vi "GetSWRevision.vi"(11 "File Path Control":path caption="File Path Control (leave blank to use Constants_Global value of EnFlo SW Folder)") -> (0 "Brief Output":string, 2 "localStatus":string, 3 "Revision":string)   [LabVIEW 2022 SP3]
doc: "This VI uses the system's installed svn (subversion) software to return the revision number of the selected folder. Leaving the selected folder blank will use the global value of \"EnFlo SW Folder\".\nThe \"Overall Revision\" is the highest revision number in the entire hierarchy, recursing upwards as well as downwards- in other words, the revision which was checked out. The \"This Folder\" data is specific to the last changes to the selected folder."
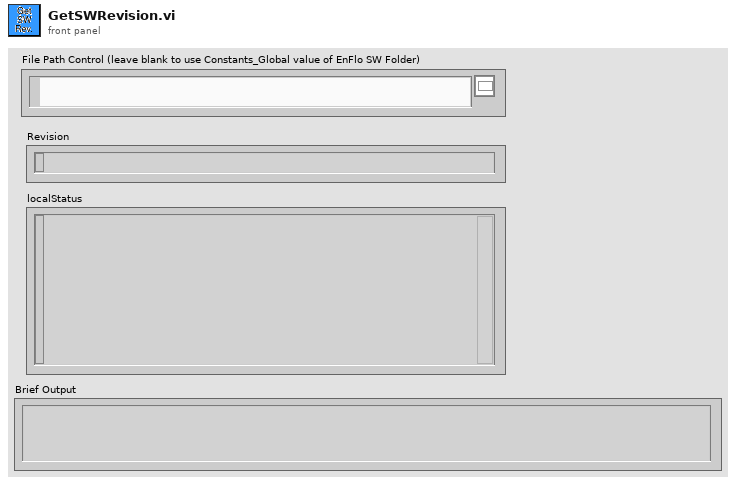
[diagram p1: front panel]
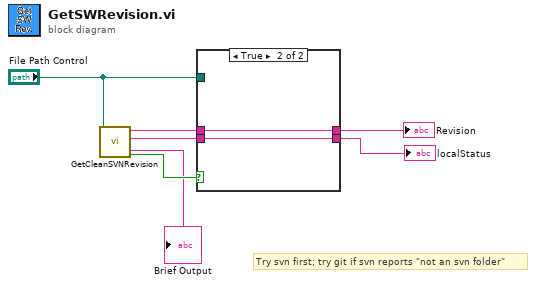
[diagram p0: block diagram]
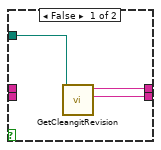
[diagram p2: hidden frame]
diagram:
  # "Try svn first; try git if svn reports \"not an svn folder\""
  n1 = call "GetCleanSVNRevision.vi"("File Path Control"="File Path Control") -> ("isSVN"=w5:bool, "svnDetails"=w7:string, "svnRevision"=w4:string, "Brief Output"=→"Brief Output":string)  [unwired: 7 in]
  n2 = case shown="True" w5 {
    tunnel: [w10 w12] -> w2
    tunnel: w7 -> [_ w12]
    tunnel: "File Path Control" -> [w9 _]
    tunnel: w4 -> [_ w11]
    tunnel: [w8 w11] -> w3
    frame False {
      n3 = call "GetCleangitRevision.vi"("File Path Control"=w9) -> ("gitDetails"=w10:string, "gitRevision"=w8:string)  [unwired: 9 in]
    }
    frame True {
    }
  }
  "Revision" <- w3
  "localStatus" <- w2
